vi "Burst.vi"(0 "RFFE RegRead Command in":refnum<class "RFFE RegRead Command.lvclass">, 1 "Bus Number":i32, 5 "instrument handle in":refnum<k15>, 11 "error in (no error)":errorcluster) -> (4 "RFFE RegRead Command out":refnum<class "RFFE RegRead Command.lvclass">, 6 "instrument handle out":refnum<k15>, 15 "error out":errorcluster)   [LabVIEW 2018, in "MIPI RFFE API.lvlib" / "RFFE RegRead Command.lvclass"]
uses:
  RFFE RegRead Command.lvclass
  C:/Users/semoore/Projects/mipi-rffe-labview-oop/Standard Command/RFFE Standard Command.lvclass
  Standard Command/RFFE Standard Command.lvclass/RFFE Standard Command.ctl
  Standard Command/Set Register Data.vi
  Standard Command/RFFE Standard Command.lvclass
  MIPI RFFE API.lvlib
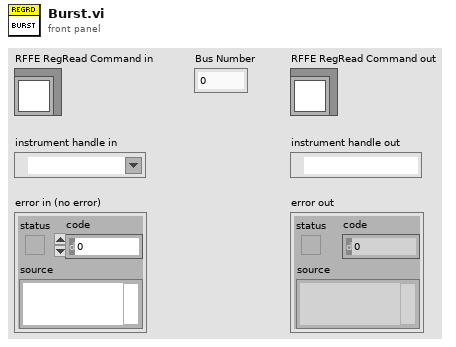
[diagram p1: front panel]
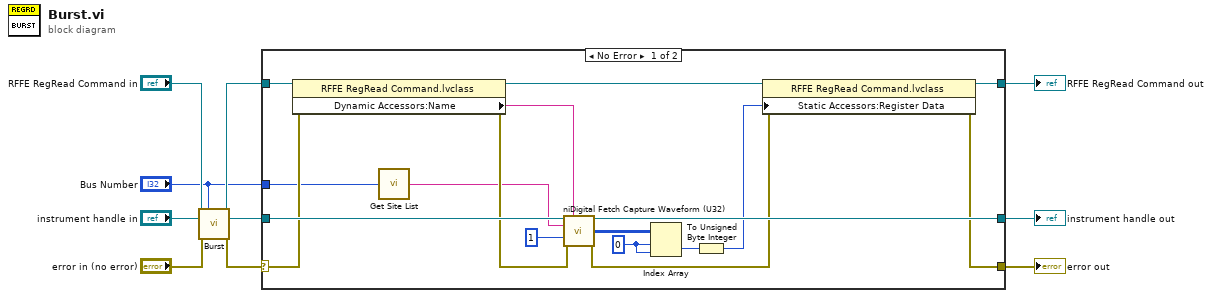
[diagram p0: block diagram]
diagram:
  n1 = call-parent "Burst.vi"("RFFE Command in"="RFFE RegRead Command in", "Bus Number"="Bus Number", "instrument handle in"="instrument handle in", "error in (no error)"="error in (no error)") -> ("RFFE Command out"=w5:refnum<class "RFFE RegRead Command.lvclass">, "instrument handle out"=w7:refnum<k15>, "error out"=w4:errorcluster)  [unwired: 9 in]
  n2 = case shown="No Error" w4 {
    selector: w4 -> [w13 w29]
    tunnel: w7 -> [w27 w28]
    tunnel: [w26 w28] -> w6
    tunnel: w5 -> [w25 w30]
    tunnel: [w20 w30] -> w3
    tunnel: [w18 w29] -> w2
    tunnel: "Bus Number" -> [w12 _]
    frame No Error {
      w16 = 0 ("index (row)")
      n3 = property class="RFFE RegRead Command.lvclass"(reference=w25, error in=w13) -> (reference out=w21:refnum<class "RFFE RegRead Command.lvclass">, error out=w23:errorcluster, "Dynamic Accessors:Name"=w24:string)
      n4 = call "Get Site List.vi"("Bus Number"=w12) -> ("Site List"=w11:string)  [unwired: 14 in]
      n5 = call <instrlib>:"niDigital Fetch Capture Waveform (U32).vi"("instrument handle"=w27, "waveform name"=w24, "site list"=w11, "samples to read"=1, "error in"=w23) -> ("instrument handle out"=w26:refnum<k15>, "data"=w17:u32[][], "error out"=w19:errorcluster)  [unwired: 8 in]
      n6 = Index Array(array=w17, index (row)=w16, index (col)=w16) -> (element=w15:u32)
      n7 = To Unsigned Byte Integer(number=w15) -> (unsigned 8bit integer=w14:u8)
      n8 = property class="RFFE RegRead Command.lvclass"(reference=w21, error in=w19, "Static Accessors:Register Data"=w14) -> (reference out=w20:refnum<class "RFFE RegRead Command.lvclass">, error out=w18:errorcluster)
    }
    frame Error {
    }
  }
  "error out" <- w2
  "RFFE RegRead Command out" <- w3
  "instrument handle out" <- w6
